vi "Do Request.vi"(7 "Processing In":refnum<class "Processing.lvclass">, 11 "LogHTTPController in":refnum<class "LogHTTPController.lvclass">) -> (0 "error out":errorcluster, 5 "Processing":refnum<class "Processing.lvclass">)   [LabVIEW 2020, in "VolatusData.lvlib" / "LogHTTPController.lvclass"]
doc: "A controller's main job is to respond to a request by generating a response. The response value must be specified by calling Set Response.vi on the Processing class that's passed through the VI otherwise an error will be generated.\n\nThere are several helpers available for common response types:\nGenerating HTML content programmatically - Create Basic Response.vi\nStreaming a file from disk - Create File Response.vi\nRedirecting the user to another URL - Create Redirect Response.vi\n\nFile responses are streamed in chunks and do not load the entire file into memory at once to send in the response which allows serving large files more efficiently."
uses:
  LogHTTPController.lvclass
  lv-http-server/HTTP Server/Processing/Processing.lvclass
  lv-http-server/HTTP Server/Processing/Processing.lvclass/Processing.ctl
  lv-http-util/HTTP Utils/Request/Request.lvclass/Request.ctl
  lv-uri/URI/URI/URI.lvclass/URI.ctl
  LogHTTPController.lvclass/LogHTTPController.ctl
  Log Status Value/Log Status Value.lvclass
  lv-http-util/HTTP Utils/Request/Get Target URI.vi
  lv-uri/URI/URI/Path String.vi
  lv-http-util/HTTP Utils/File Response/File Response.lvclass
  C:/dev/lv20CE/relink/lv-http-util/HTTP Utils/Response/Response.lvclass
  lv-http-util/HTTP Utils/Response/Response.lvclass
  Volatus/MessageQ/MessageQ.lvclass
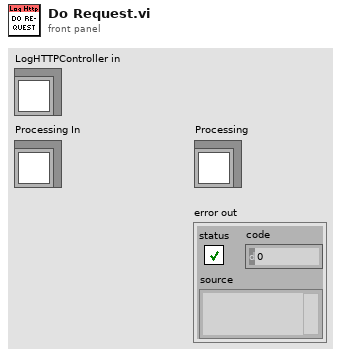
[diagram p1: front panel]
types:
  T1 = typedef "VolatusData.lvlib/Log Status.ctl" = cluster{"State":T2, "Log":string}
  T2 = typedef "VolatusData.lvlib/Logging State.ctl" = enum16{"Idle", "Starting", "Logging", "Stopping"}
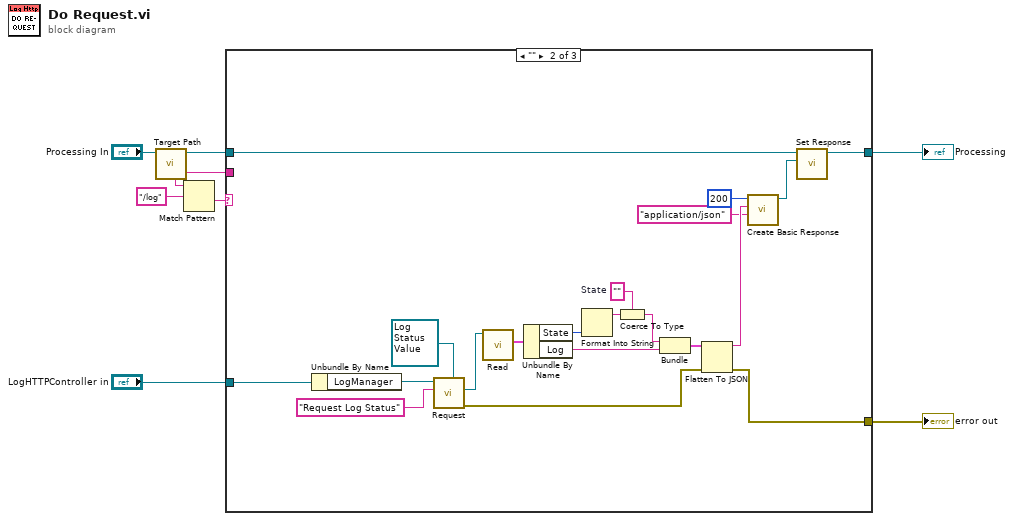
[diagram p0: block diagram]
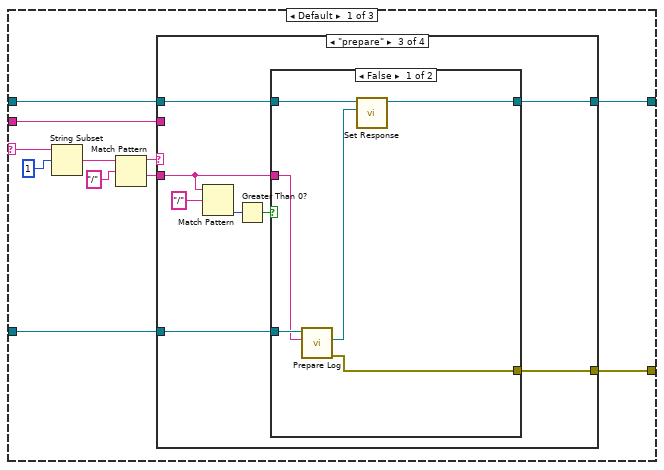
[diagram p2: hidden frame]
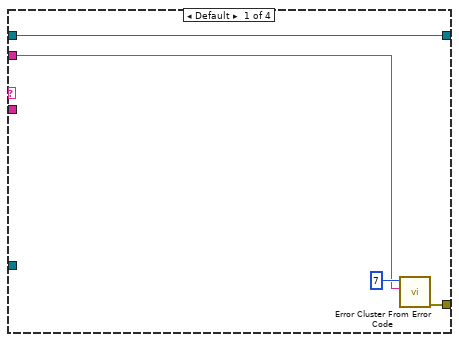
[diagram p3: hidden frame]
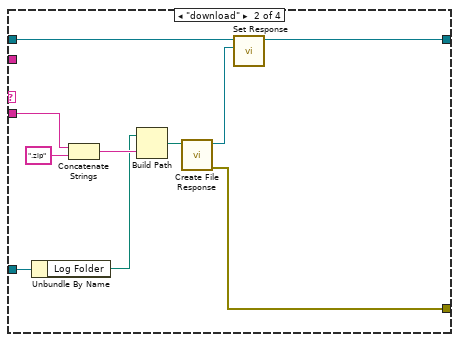
[diagram p4: hidden frame]
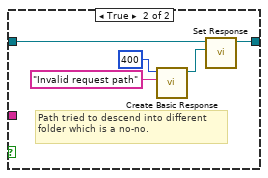
[diagram p5: hidden frame]
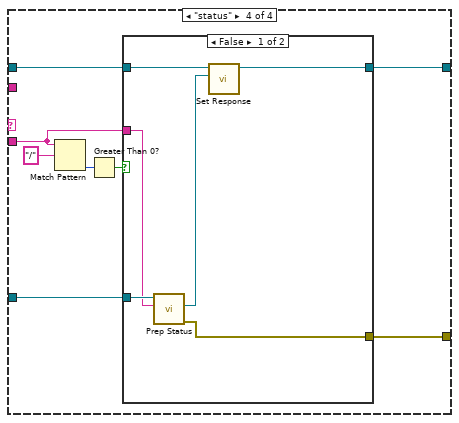
[diagram p6: hidden frame]
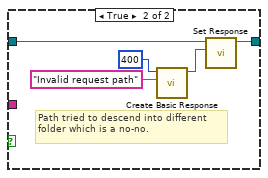
[diagram p7: hidden frame]
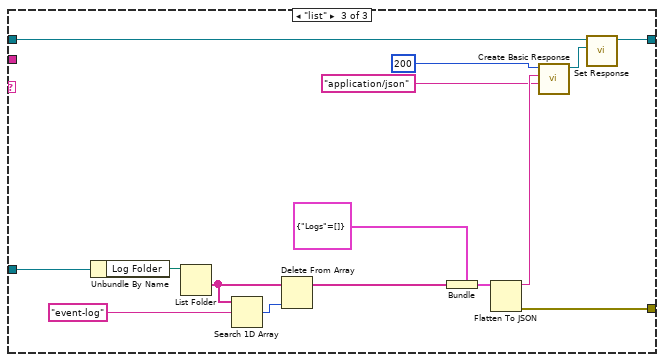
[diagram p8: hidden frame]
diagram:
  n1 = call "Target Path.vi"("Processing in"="Processing In") -> ("Processing out"=w5:refnum<class "Processing.lvclass">, "Target Path"=w3:string)  [unwired: 9 in]
  n2 = Match Pattern(string=w3, regular expression="/log") -> (after substring=w6:string)  [unwired: 1 in, 3 out]
  n3 = case shown="\"\"" w6 {
    selector: w6 -> [w11 _ _]
    tunnel: w5 -> [w16 w91 w106]
    tunnel: [w14 w75 w98] -> w4
    tunnel: w3 -> [w12 _ _]
    tunnel: [w13 w72 w102] -> w2
    tunnel: "LogHTTPController in" -> [w15 w90 w105]
    frame Default {
      n4 = String Subset(string=w11, offset (0)=1) -> (substring=w9:string)  [unwired: 1 in]
      n5 = Match Pattern(string=w9, regular expression="/") -> (before substring=w18:string, after substring=w17:string)  [unwired: 1 in, 2 out]
      n6 = case shown="\"prepare\"" w18 {
        tunnel: w17 -> [_ w31 w35 w54]
        tunnel: w16 -> [w23 w32 w38 w57]
        tunnel: w15 -> [_ w33 w36 w55]
        tunnel: [w23 w26 w37 w56] -> w14
        tunnel: [w22 w24 w34 w53] -> w13
        tunnel: w12 -> [w20 _ _ _]
        frame Default {
          n7 = call <vilib>:"Error Cluster From Error Code.vi"("error message (\"\")"=w20, "error code (0)"=7) -> ("error out"=w22:errorcluster)  [unwired: 7 in]
        }
        frame "download" {
          n8 = Unbundle By Name(w33) -> ("Log Folder"=w28:path)
          n9 = Concatenate Strings(w31, ".zip" ("string")) -> (w29:string)
          n10 = Build Path(base path=w28, name or relative path=w29) -> (appended path=w27:path)
          n11 = call "Create File Response.vi"("Path"=w27) -> ("error out"=w24:errorcluster, "File Response out"=w25:refnum<class "File Response.lvclass">)  [unwired: 9 in]
          n12 = call "Set Response.vi"("Response"=w25, "Processing in"=w32) -> ("Processing out"=w26:refnum<class "Processing.lvclass">)  [unwired: 9 in]
        }
        frame "prepare" {
          n13 = Match Pattern(string=w35, regular expression="/") -> (offset past match=w40:i32)  [unwired: 1 in, 3 out]
          n14 = Greater Than 0?(x=w40) -> (x > 0?=w39:bool)
          n15 = case shown="False" w39 {
            tunnel: w38 -> [w44 w50]
            tunnel: [w43 w48] -> w37
            tunnel: w36 -> [w47 _]
            tunnel: w35 -> [w46 _]
            tunnel: [w45 _] -> w34
            frame False {
              n16 = call "Prepare Log.vi"("Log"=w46, "LogHTTPController in"=w47) -> ("error out"=w45:errorcluster, "Response"=w42:refnum<class "Response.lvclass">)  [unwired: 7 in, 1 out]
              n17 = call "Set Response.vi"("Response"=w42, "Processing in"=w44) -> ("Processing out"=w43:refnum<class "Processing.lvclass">)  [unwired: 9 in]
            }
            frame True {
              # "Path tried to descend into different folder which is a no-no."
              n18 = call "Create Basic Response.vi"("Payload"="Invalid request path", "Status Code"=u16 400) -> ("Response out"=w49:refnum<class "Response.lvclass">)  [unwired: 8 in, 1 out]
              n19 = call "Set Response.vi"("Response"=w49, "Processing in"=w50) -> ("Processing out"=w48:refnum<class "Processing.lvclass">)  [unwired: 9 in]
            }
          }
        }
        frame "status" {
          n20 = Match Pattern(string=w54, regular expression="/") -> (offset past match=w59:i32)  [unwired: 1 in, 3 out]
          n21 = Greater Than 0?(x=w59) -> (x > 0?=w58:bool)
          n22 = case shown="False" w58 {
            tunnel: w57 -> [w63 w69]
            tunnel: [w62 w67] -> w56
            tunnel: w55 -> [w66 _]
            tunnel: w54 -> [w65 _]
            tunnel: [w64 _] -> w53
            frame False {
              n23 = call "Prep Status.vi"("Log"=w65, "LogHTTPController in"=w66) -> ("error out"=w64:errorcluster, "Response"=w61:refnum<class "Response.lvclass">)  [unwired: 7 in, 1 out]
              n24 = call "Set Response.vi"("Response"=w61, "Processing in"=w63) -> ("Processing out"=w62:refnum<class "Processing.lvclass">)  [unwired: 9 in]
            }
            frame True {
              # "Path tried to descend into different folder which is a no-no."
              n25 = call "Create Basic Response.vi"("Payload"="Invalid request path", "Status Code"=u16 400) -> ("Response out"=w68:refnum<class "Response.lvclass">)  [unwired: 8 in, 1 out]
              n26 = call "Set Response.vi"("Response"=w68, "Processing in"=w69) -> ("Processing out"=w67:refnum<class "Processing.lvclass">)  [unwired: 9 in]
            }
          }
        }
      }
    }
    frame "" {
      w81 = ""  # State
      n27 = Unbundle By Name(w90) -> ("LogManager"=w89:refnum<class "MessageQ.lvclass">)
      n28 = call "Request.vi"("Response Type (None)"=refnum<class "Log Status Value.lvclass"> refnum ("VolatusData:Log Status Value.lvclass"), "ID"="Request Log Status", "MessageQ in"=w89) -> ("error out"=w73:errorcluster, "Response"=w86:refnum<class "Log Status Value.lvclass">)  [unwired: 6 in, 1 out]
      n29 = call "Read.vi"("Log Status Value in"=w86) -> ("Log Status"=w85:T1)  [unwired: 10 in]
      n30 = Unbundle By Name(w85) -> ("State"=w84:T2, "Log"=w80:string)
      n31 = Format Into String(w84) -> (resulting string=w83:string)  [unwired: 3 in, 1 out]
      n32 = Coerce To Type(0:w83, 1:w81) -> (2:w82:string)
      n33 = Bundle("State"=w82, "Log"=w80) -> (w79:cluster{"State":string, "Log":string})  [unwired: 1 in]
      n34 = Flatten To JSON(anything=w79, error in (no error)=w73) -> (JSON string=w78:string, 11:w72:errorcluster)  [unwired: 1 in]
      n35 = call "Create Basic Response.vi"("Content-Type (text/plain)"="application/json", "Payload"=w78, "Status Code"=u16 200) -> ("Response out"=w74:refnum<class "Response.lvclass">)  [unwired: 7 in, 1 out]
      n36 = call "Set Response.vi"("Response"=w74, "Processing in"=w91) -> ("Processing out"=w75:refnum<class "Processing.lvclass">)  [unwired: 9 in]
    }
    frame "list" {
      n37 = Unbundle By Name(w105) -> ("Log Folder"=w96:path)
      n38 = List Folder(path=w96) -> (folder names=w95:string[])  [unwired: 3 in, 3 out]
      n39 = Search 1D Array(1D array=w95, element="event-log") -> (index of element=w92:i32)  [unwired: 1 in]
      n40 = Delete From Array(array=w95, index=w92) -> (array with subset deleted=w93:string[])  [unwired: 1 in, 1 out]
      n41 = Bundle(cluster=cluster{"Logs":string[]} {"Logs"=[]}, "Logs"=w93) -> (w103:cluster{"Logs":string[]})
      n42 = Flatten To JSON(anything=w103) -> (JSON string=w101:string, 11:w102:errorcluster)  [unwired: 2 in]
      n43 = call "Create Basic Response.vi"("Content-Type (text/plain)"="application/json", "Payload"=w101, "Status Code"=u16 200) -> ("Response out"=w97:refnum<class "Response.lvclass">)  [unwired: 7 in, 1 out]
      n44 = call "Set Response.vi"("Response"=w97, "Processing in"=w106) -> ("Processing out"=w98:refnum<class "Processing.lvclass">)  [unwired: 9 in]
    }
  }
  "error out" <- w2
  "Processing" <- w4
